vi "开启关闭时间.vi"(6 "计算参数 in":T2, 7 "输入参数 in":T1, 8 "进口压力信号 in":dbl[](array[numeric]), 9 "行程 in":dbl[](array[numeric])) -> (0 "计算参数 out":T2, 1 "输入参数 out":T1, 2 "进口压力信号 out":dbl[](array[numeric]), 3 "行程 out":dbl[](array[numeric]), 4 "Waveform Graph":cluster{dbl, dbl, dbl[][]}(graph))   [LabVIEW 2013]
doc: "此程序计算开启关闭时间\nCL=tv2-tv1\nOP=ts2-ts1"
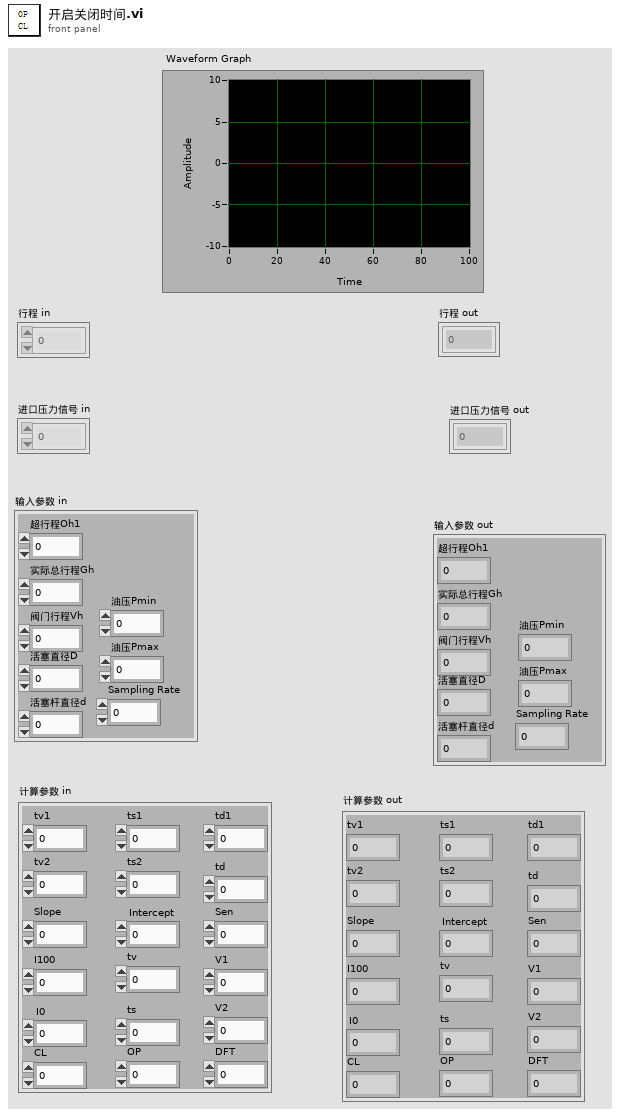
[diagram p1: front panel]
types:
  T1 = cluster{"超行程Oh1":dbl, "实际总行程Gh":dbl, "阀门行程Vh":dbl, "活塞直径D":dbl, "活塞杆直径d":dbl, "油压Pmin":dbl, "油压Pmax":dbl, "Sampling Rate":dbl}
  T2 = cluster{"tv1":dbl, "tv2":dbl, "tv":dbl, "ts1":dbl, "ts2":dbl, "ts":dbl, "td1":dbl, "td":dbl, "Slope":dbl, "Intercept":dbl, "I100":dbl, "I0":dbl, "Sen":dbl, "V1":dbl, "V2":dbl, "CL":dbl, "OP":dbl, "DFT":dbl}
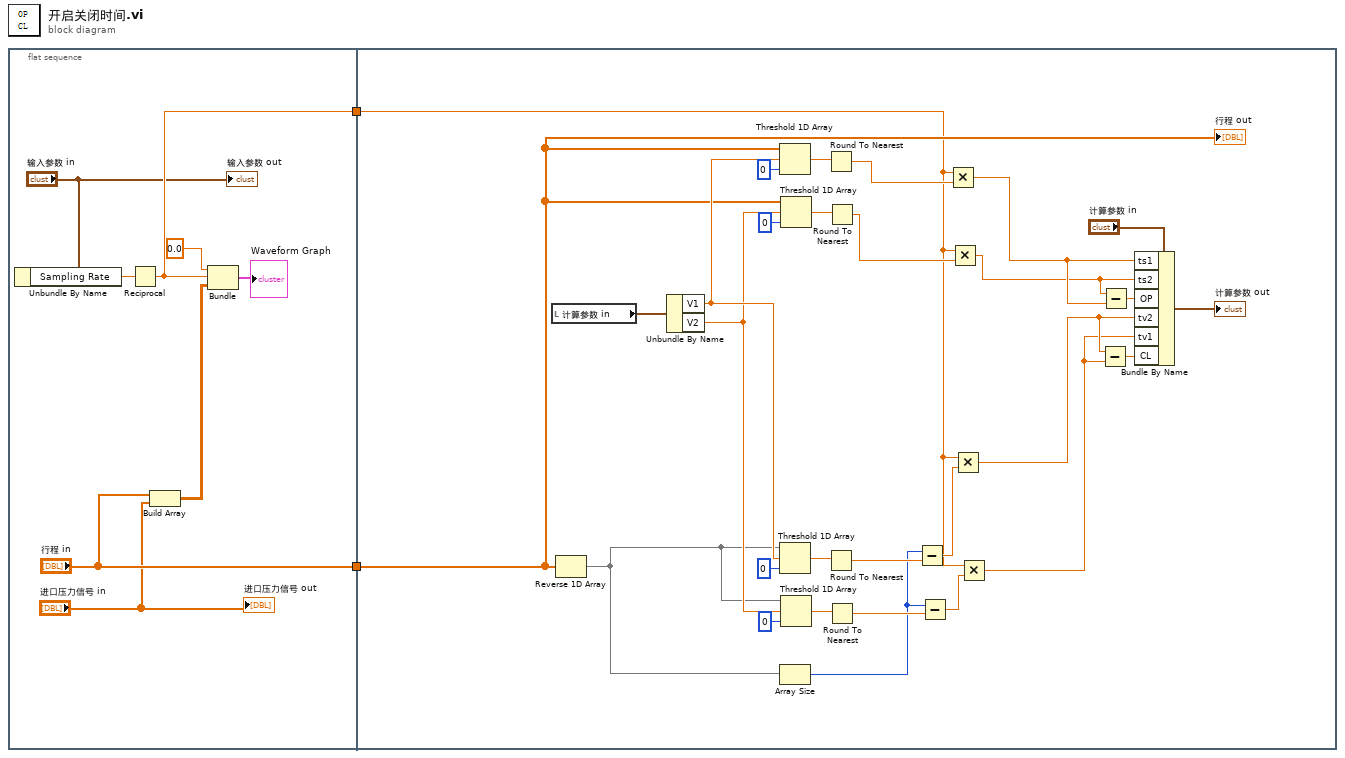
[diagram p0: block diagram]
diagram:
  n1 = flat-sequence {
    tunnel: ["行程 in"] -> w2
    tunnel: [w8] -> w1
    tunnel: w2 -> [w20]
    tunnel: w1 -> [w12]
    frame #0 {
      n2 = Unbundle By Name("输入参数 in") -> ("Sampling Rate"=w4:dbl)
      n3 = Reciprocal(x=w4) -> (1/x=w8:dbl)
      n4 = Build Array("行程 in", "进口压力信号 in") -> (w6:dbl[][])
      n5 = Bundle(0.0, w8, w6) -> (→"Waveform Graph":cluster{dbl, dbl, dbl[][]})  [unwired: 1 in]
      "输入参数 out" <- "输入参数 in"
      "进口压力信号 out" <- "进口压力信号 in"
    }
    frame #1 {
      n6 = local read "计算参数 in"() -> (w37:T2)
      n7 = Reverse 1D Array(array=w20) -> (reversed array=w24:dbl[])
      n8 = Unbundle By Name(w37) -> ("V1"=w27:dbl, "V2"=w25:dbl)
      n9 = Threshold 1D Array(1:0 ("start index (0)"), 2:w27, 3:w20) -> (0:w36:dbl)
      n10 = Threshold 1D Array(1:0 ("start index (0)"), 2:w27, 3:w24) -> (0:w31:dbl)
      n11 = Array Size(array=w24) -> (size(s)=w22:i32)
      n12 = Threshold 1D Array(1:0 ("start index (0)"), 2:w25, 3:w20) -> (0:w35:dbl)
      n13 = Threshold 1D Array(1:0 ("start index (0)"), 2:w25, 3:w24) -> (0:w30:dbl)
      n14 = Round To Nearest(number=w36) -> (nearest integer value=w19:dbl)
      n15 = Round To Nearest(number=w31) -> (nearest integer value=w26:dbl)
      n16 = Round To Nearest(number=w35) -> (nearest integer value=w16:dbl)
      n17 = Round To Nearest(number=w30) -> (nearest integer value=w23:dbl)
      n18 = Subtract(x=w22, y=w26) -> (x-y=w15:dbl)
      n19 = Subtract(x=w22, y=w23) -> (x-y=w11:dbl)
      n20 = Multiply(x=w12, y=w19) -> (x*y=w18:dbl)
      n21 = Multiply(x=w12, y=w16) -> (x*y=w17:dbl)
      n22 = Multiply(x=w12, y=w15) -> (x*y=w14:dbl)
      n23 = Multiply(x=w12, y=w11) -> (x*y=w13:dbl)
      n24 = Subtract(x=w14, y=w13) -> (x-y=w21:dbl)
      n25 = Subtract(x=w17, y=w18) -> (x-y=w32:dbl)
      n26 = Bundle By Name(cluster="计算参数 in", "ts1"=w18, "ts2"=w17, "OP"=w32, "tv2"=w14, "tv1"=w13, "CL"=w21) -> (→"计算参数 out":T2)
      "行程 out" <- w20
    }
  }
